vi "frequencysignals2.vi"(0 "Offset":dbl(knob) scale=-10.0..10.0, 2 "Reset Signal":bool, 5 "Frequency":dbl(knob)=10.1 scale=0.0..500.0, 7 "Amplitude":dbl(knob)=1.0 scale=0.0..10.0 scale format="%#.1f", 9 "Phase":dbl(knob) scale=0.0..10.0, 11 "error in (no error)":errorcluster) -> (4 "Sine":dynamicdata(graph), 15 "error out":errorcluster)   [LabVIEW 2015]
doc: "Simulates a sine wave, square wave, triangle wave, sawtooth wave, or noise signal.\n--------------------\n\nThis Express VI is configured as follows:\n\nSignal Type: Sine\nFrequency: 10,1 Hz\nAmplitude: 1\nPhase: 0\nOffset: 0\nSampling Rate: 1000 Hz\nNumber of Samples: 100 (Automatic)\nTiming: Run as fast as possible\nTimestamps: Relative"
panel:
  in  "Noise":bool
  in  "Noise Ring":u16(ring) items=["Uniform White Noise", "Gaussian White Noise", "Periodic Random Noise", "Gamma Noise", "Poisson Noise", "Binomial Noise", "Bernoulli Noise", "MLS Sequence "]
  in  "Generate":T1(ring)
  in  "stop":bool
  in  "Trials":i32=1
  in  "Seed Number":dbl=-1.0
  in  "Noise amplitude":dbl=0.6 step=0.1
  in  "Duty Cycle (%)":dbl(knob)=50.0 scale=0.0..10.0
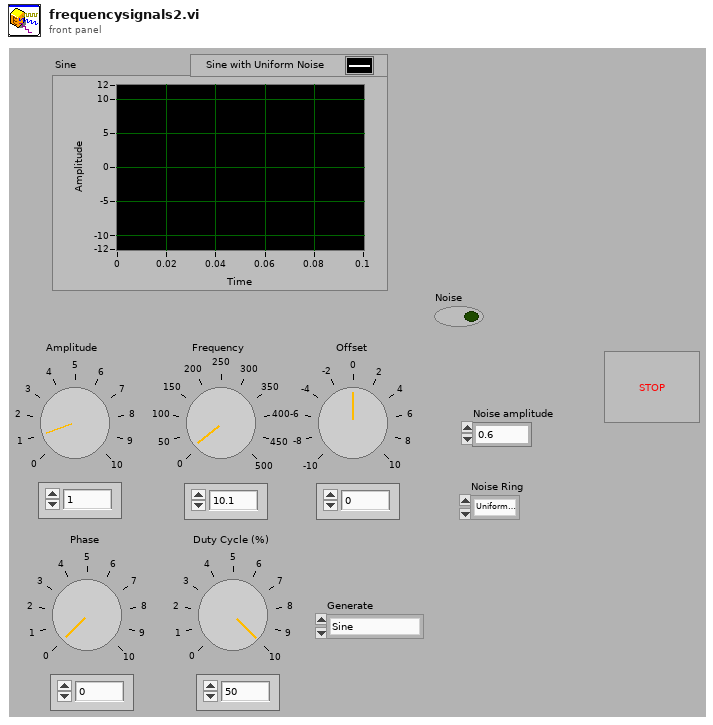
[diagram p1: front panel]
types:
  T1 = enum16{"Sine", "Square", "Triangle", "Sawtooth", "DC"}
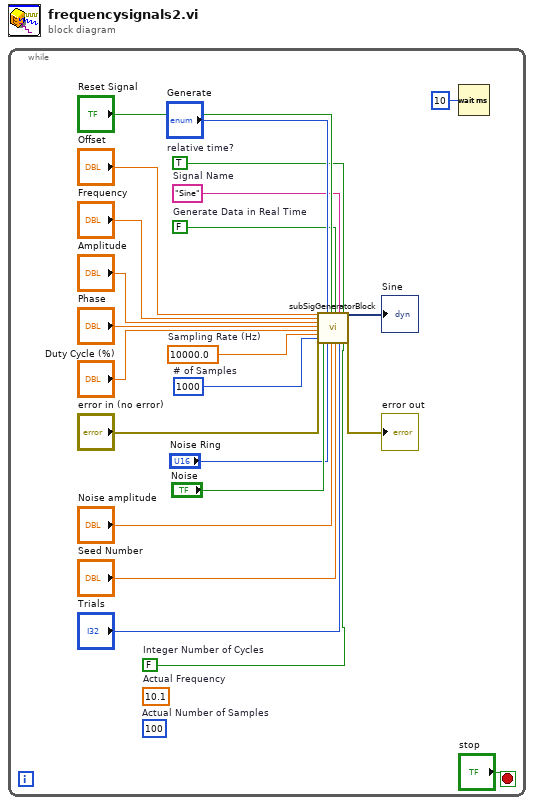
[diagram p0: block diagram]
diagram:
  n1 = while {
    stop <- "stop" stop-if-true
    (unwired) 10.1  # Actual Frequency
    (unwired) 100  # Actual Number of Samples
    w3 = FALSE  # Integer Number of Cycles
    w11 = TRUE  # relative time?
    w12 = "Sine"  # Signal Name
    w13 = FALSE  # Generate Data in Real Time
    w17 = 1000  # # of Samples
    w19 = 10000.0  # Sampling Rate (Hz)
    n2 = call <vilib>:"subSigGeneratorBlock.vi"("Offset"="Offset", "Frequency"="Frequency", "Amplitude"="Amplitude", "Phase"="Phase", "Duty Cycle (%)"="Duty Cycle (%)", "Sampling Rate (Hz)"=w19, "# of Samples"=w17, "error in (no error)"="error in (no error)", "Noise"="Noise", "Generate"="Generate", "Noise Ring"="Noise Ring", "Reset Signal"="Reset Signal", "Noise Amplitude"="Noise amplitude", "Generate Data in Real Time"=w13, "Seed Number"="Seed Number", "Signal Name"=w12, "trials"="Trials", "relative time?"=w11, "Integer Number of Cycles"=w3) -> ("Signal"=→"Sine":dynamicdata, "error out"=→"error out":errorcluster)  [unwired: 7 in]
    n3 = Wait (ms)(milliseconds to wait=u32 10) -> ()  [unwired: 1 out]
  }
